vi "Find.vi"(8 "Error In":errorcluster, 10 "Key":string, 11 "Map In":refnum<class "Map.lvclass">) -> (0 "Error Out":errorcluster, 1 "Found?":bool, 2 "Value":refnum<class "Abstract.lvclass">, 3 "Map Out":refnum<class "Map.lvclass">)   [LabVIEW 2018, in "Toolkit.lvlib" / "Data.lvlib" / "Map.lvclass"]
uses:
  Map.lvclass
  Abstract/Abstract.lvclass
  Null/Null.lvclass
  D:/Users/cfield/Code/Field R&D Services/Mustache/trunk/src/Toolkit/Data/Abstract/Abstract.lvclass
  Map.lvclass/Map.ctl
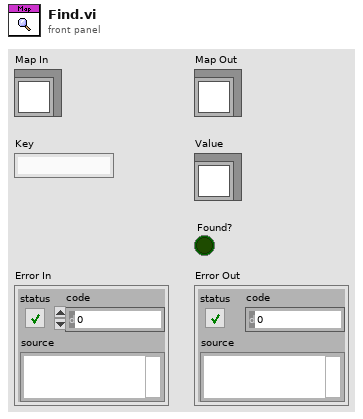
[diagram p1: front panel]
types:
  T1 = cluster{"Key":string, "Value":refnum<class "Abstract.lvclass">}[]
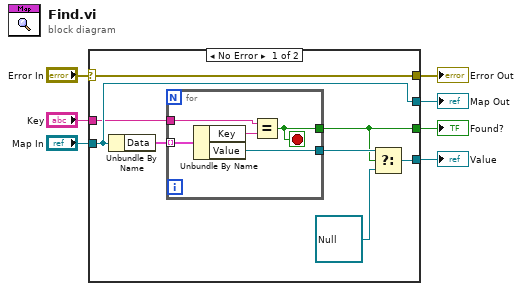
[diagram p0: block diagram]
diagram:
  n1 = case shown="No Error" "Error In" {
    selector: "Error In" -> [w12 w22]
    tunnel: "Map In" -> [w15 w21]
    tunnel: [w12 w22] -> w5
    tunnel: [w15 w21] -> w4
    tunnel: "Key" -> [w13 _]
    tunnel: [w9 _] -> w2
    tunnel: [w8 _] -> w1
    frame No Error {
      n2 = Unbundle By Name(w15) -> ("Data"=w14:T1)
      n3 = for {
        tunnel: w14 -> [w20] mode=indexing
        tunnel: w13 -> [w19]
        tunnel: [w17] -> w11
        tunnel: [w16] -> w8
        stop <- w16 stop-if-true
        n4 = Unbundle By Name(w20) -> ("Key"=w18:string, "Value"=w17:refnum<class "Abstract.lvclass">)
        n5 = Equal?(x=w19, y=w18) -> (x = y?=w16:bool)
      }
      n6 = Select(t=w11, s=w8, f=refnum<class "Null.lvclass"> refnum ("Toolkit.lvlib:Data.lvlib:Null.lvclass")) -> (s? t:f=w9:refnum<class "Abstract.lvclass">)
    }
    frame Error {
    }
  }
  "Error Out" <- w5
  "Map Out" <- w4
  "Value" <- w2
  "Found?" <- w1
